vi "new value.vi"(4 "Label":T2="__init__", 6 "operation":T1, 7 "Previous":variant, 8 "error in (no error)":errorcluster, 9 "Other":variant, 10 "data":T3, 11 "Value in":refnum<class "Value.lvclass">) -> (0 "error out":errorcluster, 3 "Value out":refnum<class "Value.lvclass">)   [LabVIEW 2023, in "LabGRAD.lvlib" / "Value.lvclass"]
uses:
  Value.lvclass
  UiObjects/numeric value control.ctl
  UiObjects/string control.ctl
  operation.ctl
  Value.lvclass/Value.ctl
  UiObjects/UiObjects.lvclass
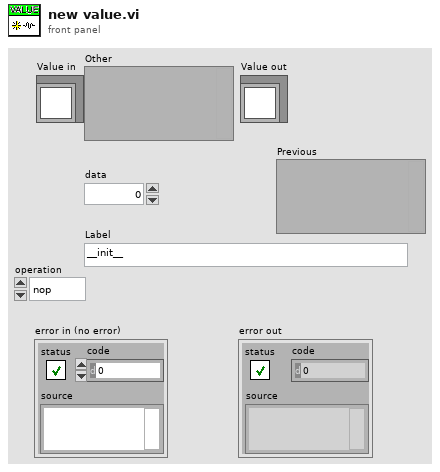
[diagram p1: front panel]
types:
  T1 = typedef "LabGRAD.lvlib/Value.lvclass/operation.ctl" = enum16{"nop", "add", "subtract", "power", "multiply", "divide", "tanh"}
  T2 = typedef "UiObjects.lvlib/UiObjects.lvclass/string control.ctl" = string
  T3 = typedef "UiObjects.lvlib/UiObjects.lvclass/numeric value control.ctl" = dbl
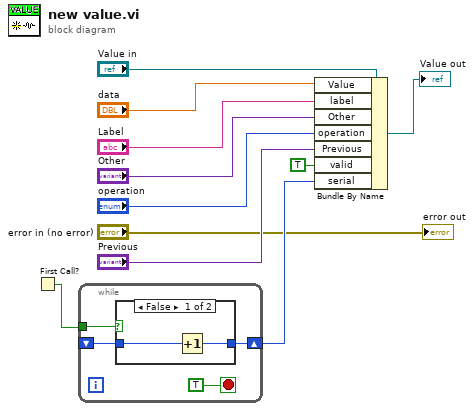
[diagram p0: block diagram]
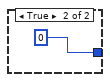
[diagram p2: hidden frame]
diagram:
  n1 = First Call?() -> (First Call?: T/F=w3:bool)
  n2 = while {
    shift-right: [w15] -> w4
    shift-left: _ -> [w14]
    tunnel: w3 -> [w12]
    stop <- TRUE stop-if-true
    n3 = case shown="False" w12 {
      tunnel: [w16 u32 0 ("serial")] -> w15
      tunnel: w14 -> [w17 _]
      frame False {
        n4 = Increment(x=w17) -> (x+1=w16:u32)
      }
      frame True {
      }
    }
  }
  n5 = Bundle By Name(cluster="Value in", "Value"="data", "label"="Label", "Other"="Other", "operation"="operation", "Previous"="Previous", "valid"=TRUE, "serial"=w4) -> (→"Value out":refnum<class "Value.lvclass">)
  "error out" <- "error in (no error)"
